vi "Default Position.vi"(0 "Selected Doc[]":refnum<class "Document.lvclass">[](array[class]), 5 "Position[]":T1[](array[typedef]), 11 "error in":errorcluster) -> (4 "Selected Doc[]":refnum<class "Document.lvclass">[](array[class]), 6 "Position[]":T1[](array[typedef]), 15 "error Out":errorcluster)   [LabVIEW 2016, in "LV MDI.lvclass"]
uses:
  LV MDI.lvclass
  TypeDefs/Set Position.ctl
  Document/Document.lvclass
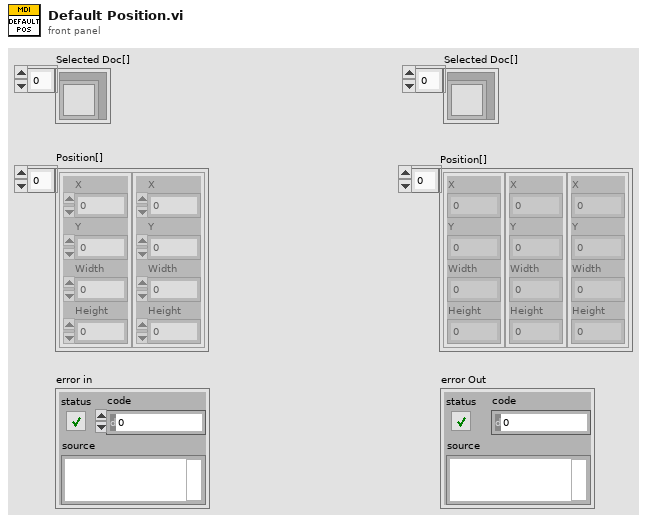
[diagram p1: front panel]
types:
  T1 = typedef "LV MDI.lvclass/Set Position.ctl" = cluster{"X":i32, "Y":i32, "Width":i32, "Height":i32}
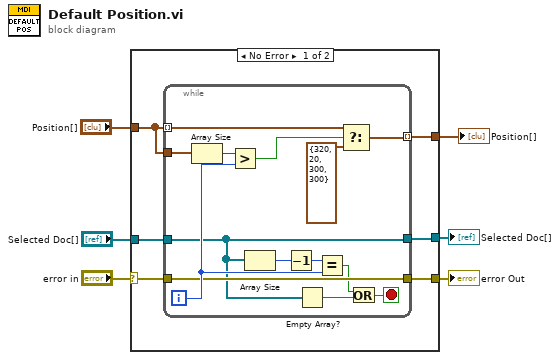
[diagram p0: block diagram]
diagram:
  n1 = case shown="No Error" "error in" {
    selector: "error in" -> [w9 w29]
    tunnel: [w12 w28] -> w6
    tunnel: "Position[]" -> [w11 w28]
    tunnel: "Selected Doc[]" -> [w10 w27]
    tunnel: [w8 w29] -> w2
    tunnel: [w7 w27] -> w1
    frame No Error {
      n2 = while {
        tunnel: w10 -> [w14]
        tunnel: w11 -> [w22] mode=indexing
        tunnel: [w20] -> w12 mode=indexing
        tunnel: w11 -> [w25]
        tunnel: w9 -> [w18]
        tunnel: [w18] -> w8
        tunnel: [w14] -> w7
        i -> [w19]
        stop <- w16 stop-if-true
        n3 = Array Size(array=w25) -> (size(s)=w24:i32)
        n4 = Greater?(x=w24, y=w19) -> (0:w23:bool)
        n5 = Array Size(array=w14) -> (size(s)=w26:i32)
        n6 = Decrement(x=w26) -> (x-1=w17:i32)
        n7 = Empty Array?(array=w14) -> (empty?=w13:bool)
        n8 = Equal?(x=w17, y=w19) -> (x = y?=w15:bool)
        n9 = Select(t=w22, s=w23, f=T1 {"X"=320, "Y"=20, "Width"=300, "Height"=300}) -> (s? t:f=w20:T1)
        n10 = Or(x=w15, y=w13) -> (x .or. y?=w16:bool)
      }
    }
    frame Error {
    }
  }
  "Position[]" <- w6
  "error Out" <- w2
  "Selected Doc[]" <- w1
